vi "AutoPathLogic.vi"(8 "YCoordinates":dbl[](array[numeric]), 9 "XCoordinates":dbl[](array[numeric]), 10 "Y":dbl, 11 "X":dbl) -> (3 "Angle":dbl)   [LabVIEW 2017]
uses:
  <vilib>/Analysis/polynomials.llb/Polynomial Plot (Range).vi
  <vilib>/Analysis/polynomials.llb/Scalar Polynomial Evaluation (DBL).vi
  <vilib>/Analysis/NI_AALPro.lvlib
panel:
  out "AutoPathProgress":cluster{dbl[], "P(A)":dbl[]}(graph)
  out "PlannedAutoPath":cluster{dbl[], "P(A)":dbl[]}(graph)
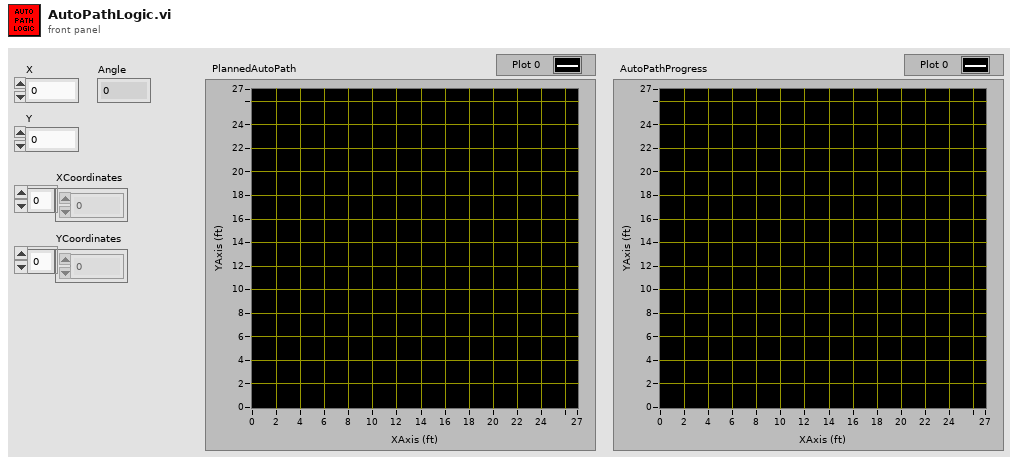
[diagram p1: front panel]
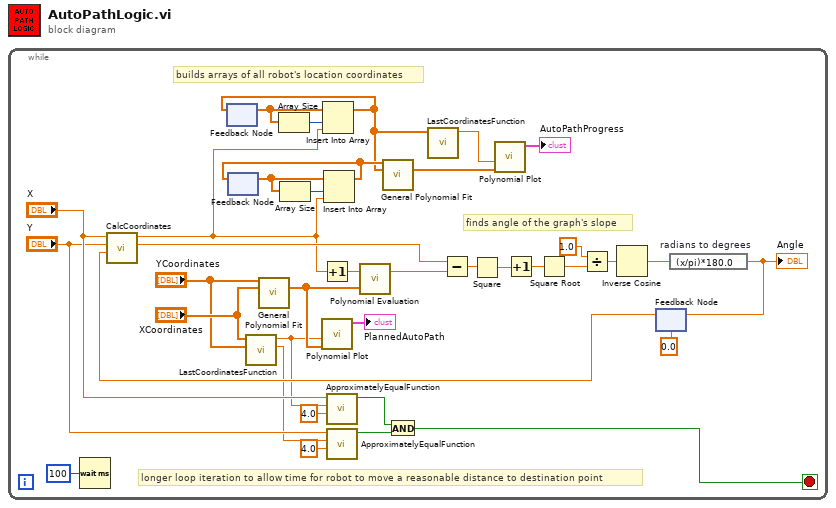
[diagram p0: block diagram]
diagram:
  n1 = while {
    stop <- w1 stop-if-true
    # "builds arrays of all robot's location coordinates"
    # "longer loop iteration to allow time for robot to move a reasonable distance to destination point"
    # "finds angle of the graph's slope"
    n2 = Wait (ms)(milliseconds to wait=u32 100) -> ()  [unwired: 1 out]
    n3 = feedback #1() -> (w22:dbl[])  [unwired: 1 in]
    n4 = feedback #2() -> (w19:dbl[])  [unwired: 1 in]
    n5 = call "LastCoordinatesFunction.vi"("YArray"="YCoordinates", "XArray"="XCoordinates") -> ("LastYCoordinate"=w6:dbl, "LastXCoordinate"=w8:dbl)  [unwired: 8 in]
    n6 = call <vilib>:"General Polynomial Fit.vi"("Y"="YCoordinates", "X"="XCoordinates") -> ("Polynomial Coefficients"=w26:dbl[])  [unwired: 10 in, 3 out]
    n7 = Array Size(array=w22) -> (size(s)=w20:i32)
    n8 = Array Size(array=w19) -> (size(s)=w18:i32)
    n9 = call-poly <vilib>:"Polynomial Plot.vi"("P(x)"=w26, "end"=w8) -> ("polynomial plot"=→"PlannedAutoPath":cluster{"Ramp Pattern":dbl[], "P(A)":dbl[]})  [unwired: 8 in, 1 out]
    n10 = call "ApproximatelyEqualFunction.vi"("Margin"=4.0, "Setpoint"=w8, "Variable"="X") -> ("t/f"=w3:bool)  [unwired: 8 in]
    n11 = call "ApproximatelyEqualFunction.vi"("Margin"=4.0, "Setpoint"=w6, "Variable"="Y") -> ("t/f"=w2:bool)  [unwired: 8 in]
    n12 = And(x=w3, y=w2) -> (x .and. y?=w1:bool)
    n13 = feedback #3(0.0) -> (w27:dbl)
    n14 = call "CalcCoordinates.vi"("SwerveAngles"=w27, "Y"="Y", "X"="X") -> ("Y'"=w21:dbl, "X'"=w17:dbl)  [unwired: 7 in]
    n15 = Increment(x=w17) -> (x+1=w30:dbl)
    n16 = Insert Into Array(array=w22, index=w20, new element=w17) -> (w13:dbl[])
    n17 = feedback-in #1(w13) -> ()
    n18 = Insert Into Array(array=w19, index=w18, new element=w17) -> (w16:dbl[])
    n19 = feedback-in #2(w16) -> ()
    n20 = call-poly <vilib>:"Polynomial Evaluation.vi"("P(x)"=w26, "a"=w30) -> ("P(a)"=w29:dbl)  [unwired: 1 out]
    n21 = call <vilib>:"General Polynomial Fit.vi"("Y"=w16, "X"=w13) -> ("Polynomial Coefficients"=w14:dbl[])  [unwired: 10 in, 3 out]
    n22 = call "LastCoordinatesFunction.vi"("XArray"=w13) -> ("LastXCoordinate"=w12:dbl)  [unwired: 9 in, 1 out]
    n23 = Subtract(x=w21, y=w29) -> (x-y=w37:dbl)
    n24 = Square(x=w37) -> (x^2=w36:dbl)
    n25 = call-poly <vilib>:"Polynomial Plot.vi"("P(x)"=w14, "end"=w12) -> ("polynomial plot"=→"AutoPathProgress":cluster{"Ramp Pattern":dbl[], "P(A)":dbl[]})  [unwired: 8 in, 1 out]
    n26 = Increment(x=w36) -> (x+1=w35:dbl)
    n27 = Square Root(x=w35) -> (sqrt(x)=w34:dbl)
    n28 = Divide(x=1.0, y=w34) -> (x/y=w33:dbl)
    n29 = Inverse Cosine(1:w33) -> (0:w25:dbl)
    n30 = expression code="(x/pi)*180.0" "radians to degrees"(w25) -> (w32:dbl)
    "Angle" <- w32
    n31 = feedback-in #3(w32) -> ()
  }
